vi "Raw Data Stream Receiver.vi"(8 "error in (no error)":errorcluster, 10 "Raw Stream Ctrl":refnum<notifier>) -> (0 "error out":errorcluster)   [LabVIEW 2015, in "Tool Module.lvlib"]
doc: "<b>Note:</b> This VI was modified by the <b>Validate DQMH Module</b> tool to turn off automatic error handling."
uses:
  Tool Module.lvlib
  _HS Data Stream Params Cluster--typedef.ctl
  _HS Data Stream SM enum--typedef.ctl
  Tool Interface/GLOB - Configuration Options.vi
  Tool Interface/Tool Interface.lvlib
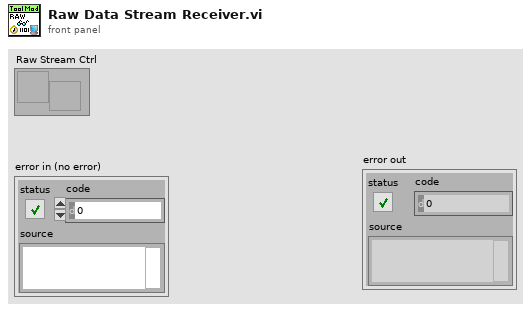
[diagram p1: front panel]
types:
  T1 = typedef "Tool Module.lvlib/_HS Data Stream Params Cluster--typedef.ctl" = cluster{"Raw Data Stream Loop cmd":T2, "Data Array DVR ref":refnum<data-value>, "HS Sample Data notifier":refnum<notifier>, "Block Count Notifier":refnum<notifier>}
  T2 = typedef "Tool Module.lvlib/_HS Data Stream SM enum--typedef.ctl" = enum16{"Idle", "Receive HS Data", "Close Connection"}
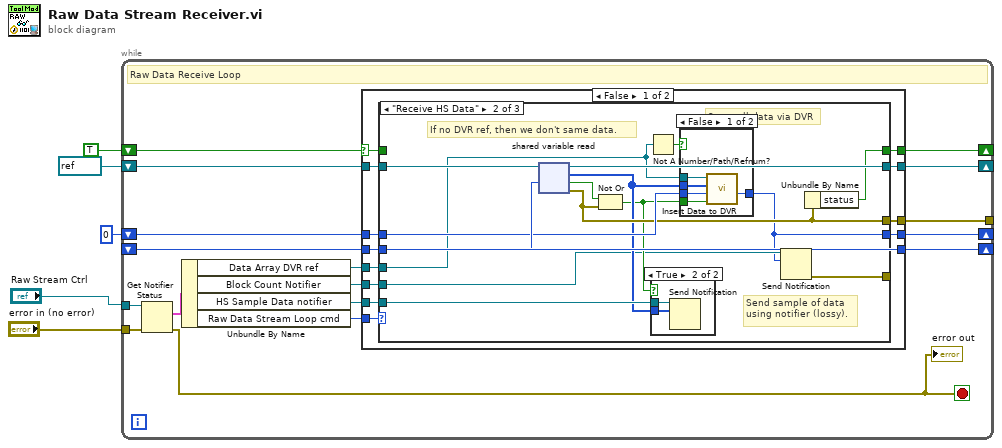
[diagram p0: block diagram]
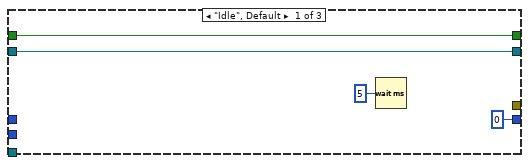
[diagram p2: hidden frame]
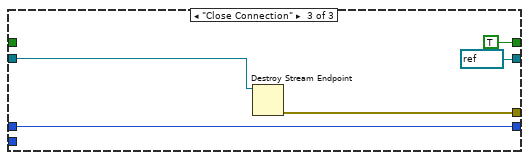
[diagram p5: hidden frame]
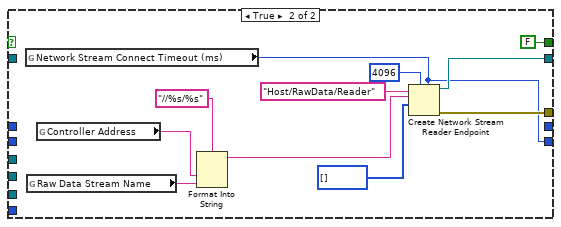
[diagram p6: hidden frame]
diagram:
  n1 = while {
    shift-right: [w21] -> _
    shift-left: TRUE -> [w22]
    shift-right: [w20] -> _
    shift-left: refnum<k21> refnum ("reader name") -> [w19]
    shift-right: [w18] -> _
    shift-left: _ -> [w17]
    tunnel: "Raw Stream Ctrl" -> [w16]
    tunnel: "error in (no error)" -> [w14]
    shift-right: [w12] -> _
    shift-left: u32 0 -> [w13]
    tunnel: [w7] -> _
    stop <- w15 stop-if-true
    # "Raw Data Receive Loop"
    n2 = Get Notifier Status(notifier=w16, error in (no error)=w14) -> (current notification=w11:T1, error out=w15:errorcluster)  [unwired: 3 out]
    "error out" <- w15
    n3 = Unbundle By Name(w11) -> ("Data Array DVR ref"=w8:refnum<data-value>, "Block Count Notifier"=w6:refnum<notifier>, "HS Sample Data notifier"=w9:refnum<notifier>, "Raw Data Stream Loop cmd"=w10:T2)
    n4 = case shown="False" w22 {
      selector: w22 -> [w32 _]
      tunnel: [w34 FALSE ("status")] -> w21
      tunnel: w10 -> [w33 _]
      tunnel: [w31 w77] -> w7
      tunnel: [w29 w76] -> w20
      tunnel: w19 -> [w30 _]
      tunnel: [w28 w67] -> w18
      tunnel: w17 -> [w28 _]
      tunnel: w13 -> [w27 _]
      tunnel: [w26 _] -> w12
      tunnel: w9 -> [w25 _]
      tunnel: w8 -> [w24 _]
      tunnel: w6 -> [w23 _]
      frame False {
        n5 = case shown="\"Receive HS Data\"" w33 {
          tunnel: [w37 w44 TRUE] -> w34
          tunnel: w32 -> [w37 _ _]
          tunnel: [_ w50 w62] -> w31
          tunnel: w30 -> [w36 w45 w65]
          tunnel: [w36 w46 refnum<k21> refnum ("reader name")] -> w29
          tunnel: w28 -> [_ w52 _]
          tunnel: w27 -> [_ w51 w63]
          tunnel: [u32 0 ("Sample Count out") w42 w63] -> w26
          tunnel: w25 -> [_ w49 _]
          tunnel: w24 -> [_ w40 _]
          tunnel: w23 -> [_ w43 _]
          tunnel: [_ w41 _] -> _
          frame "Idle", Default {
            n6 = Wait (ms)(milliseconds to wait=u32 5) -> ()  [unwired: 1 out]
          }
          frame "Receive HS Data" {
            # "If no DVR ref, then we don't same data."
            # "Store all data via DVR"
            # "Send sample of data\nusing notifier (lossy)."
            n7 = shared-variable-read(w45, w52) -> (w46:refnum<k21>, w50:errorcluster, w53:bool, w48:u32[])  [unwired: 1 in]
            n8 = Not Or(1:w50, 2:w53) -> (0:w47:bool)
            n9 = Not A Number/Path/Refnum?(number/path/refnum=w40) -> (NaN/Path/Refnum?=w39:bool)
            n10 = case shown="True" w47 {
              tunnel: w49 -> [_ w61]
              tunnel: w48 -> [_ w60]
              frame False {
              }
              frame True {
                n11 = Send Notification(notification=w60, notifier=w61) -> ()  [unwired: 1 in, 2 out]
              }
            }
            n12 = case shown="False" w39 {
              tunnel: w51 -> [w58 w59]
              tunnel: w40 -> [w57 _]
              tunnel: w48 -> [w56 _]
              tunnel: w47 -> [w55 _]
              tunnel: [w54 w59] -> w42
              frame False {
                n13 = call "Insert Data to DVR.vi"("Data Available"=w55, "Sample Count"=w58, "New Data"=w56, "Probe Data Array DVR"=w57) -> ("Sample Count out"=w54:u32)  [unwired: 7 in]
              }
              frame True {
              }
            }
            n14 = Send Notification(notification=w42, notifier=w43) -> (error out=w41:errorcluster)  [unwired: 1 in, 1 out]
            n15 = Unbundle By Name(w50) -> ("status"=w44:bool)
          }
          frame "Close Connection" {
            n16 = Destroy Stream Endpoint(11:w65) -> (0:w62:errorcluster)  [unwired: 1 in]
          }
        }
      }
      frame True {
        n17 = global read "GLOB - Configuration Options.vi" "Network Stream Connect Timeout (ms)"() -> (w67:i32)
        n18 = global read "GLOB - Configuration Options.vi" "Raw Data Stream Name"() -> (w68:string)
        n19 = global read "GLOB - Configuration Options.vi" "Controller Address"() -> (w73:string)
        n20 = Format Into String(format string="//%s/%s", w73, w68) -> (resulting string=w70:string)  [unwired: 2 in, 1 out]
        n21 = Create Network Stream Reader Endpoint(5:w67, 7:4096 ("reader buffer size"), 9:u32[] [], 10:w70, 11:"Host/RawData/Reader" ("reader name")) -> (0:w77:errorcluster, 3:w76:refnum<k21>)  [unwired: 2 in]
      }
    }
  }
